vi "Get PDO Communication Parameters.vi"(8 "error in":errorcluster, 10 "Type":enum16{"TPDO", "RPDO"}(ring), 11 "EDS in":refnum<class "Electronic Datasheet.lvclass">) -> (0 "error out":errorcluster, 2 "Entries":refnum<class "OD Entry.lvclass">[](array[class]), 3 "EDS out":refnum<class "Electronic Datasheet.lvclass">)   [LabVIEW 2019, in "Electronic Datasheet.lvlib" / "Electronic Datasheet.lvclass"]
uses:
  Electronic Datasheet/Electronic Datasheet.lvclass
  Electronic Datasheet/Electronic Datasheet.lvclass/Electronic Datasheet.ctl
  Sorted Object Dictionary.lvclass
  Electronic Datasheet.lvlib
  OD Entry/OD Entry.lvclass
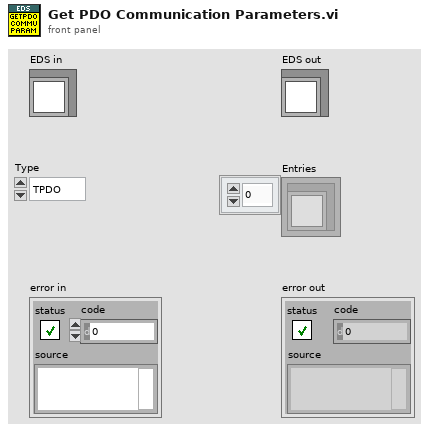
[diagram p1: front panel]
types:
  T1 = typedef "Electronic Datasheet.lvlib/Electronic Datasheet.lvclass/ObjectAttributes.ctl" = cluster{"EDS File Path":path, "Object Dict":refnum<class "Dictionary.lvclass">, "Sorted Object Dict":refnum<class "Sorted Object Dictionary.lvclass">, "Device Info":refnum<class "Device Info.lvclass">, "File Info":refnum<class "File Info.lvclass">}
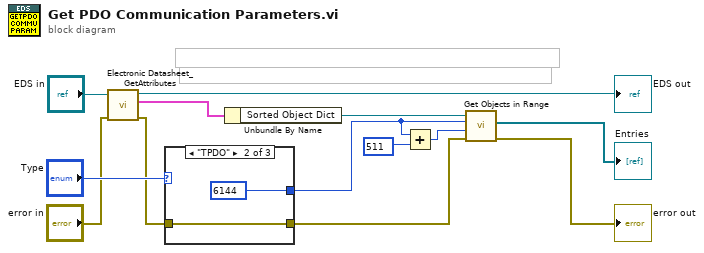
[diagram p0: block diagram]
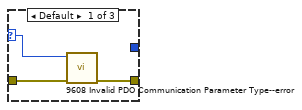
[diagram p2: hidden frame]
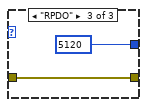
[diagram p3: hidden frame]
diagram:
  n1 = call "Electronic Datasheet_GetAttributes.vi"("Error In"="error in", "reference in"="EDS in") -> ("Error Out"=w3:errorcluster, "Data"=w7:T1, "reference out"=→"EDS out":refnum<class "Electronic Datasheet.lvclass">)  [unwired: 6 in, 1 out]
  n2 = case shown="\"TPDO\"" "Type" {
    selector: "Type" -> [w14 _ _]
    tunnel: w3 -> [w16 w18 w19]
    tunnel: [w15 w18 w19] -> w12
    tunnel: [_ u16 6144 ("Lower Bound") u16 5120 ("Lower Bound")] -> w11
    frame Default {
      n3 = call "9608 Invalid PDO Communication Parameter Type--error.vi"("error in"=w16, "Type"=w14) -> ("error out"=w15:errorcluster)  [unwired: 9 in]
    }
    frame "TPDO" {
    }
    frame "RPDO" {
    }
  }
  n4 = Unbundle By Name(w7) -> ("Sorted Object Dict"=w5:refnum<class "Sorted Object Dictionary.lvclass">)
  n5 = Add(x=w11, y=u16 511) -> (x+y=w9:u16)
  n6 = call "Get Objects in Range.vi"("error in"=w12, "Upper Bound"=w9, "Lower Bound"=w11, "Sorted Object Dictionary in"=w5) -> ("error out"=→"error out":errorcluster, "Entries"=→"Entries":refnum<class "OD Entry.lvclass">[])  [unwired: 5 in, 1 out]
